vi "Read Roles.vi"(8 "error in (no error)":errorcluster, 11 "KickPenaltyAllyPlayVSS in":refnum<class "KickPenaltyAllyPlayVSS.lvclass">) -> (0 "error out":errorcluster, 2 "Roles":T1, 3 "KickPenaltyAllyPlayVSS out":refnum<class "KickPenaltyAllyPlayVSS.lvclass">)   [LabVIEW 2020, in "KickPenaltyAllyPlayVSS.lvclass"]
uses:
  KickPenaltyAllyPlayVSS.lvclass
  NormalAttackerRoleVSS_class/NormalAttackerRoleVSS.lvclass
  HaltRole_class/HaltRole.lvclass
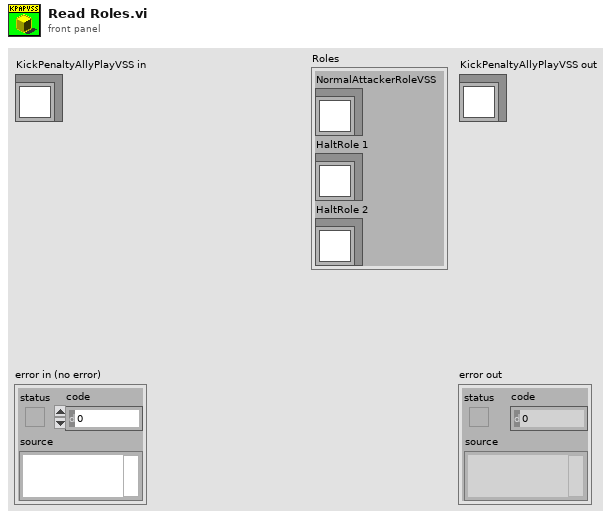
[diagram p1: front panel]
types:
  T1 = cluster{"NormalAttackerRoleVSS":refnum<class "NormalAttackerRoleVSS.lvclass">, "HaltRole 1":refnum<class "HaltRole.lvclass">, "HaltRole 2":refnum<class "HaltRole.lvclass">}
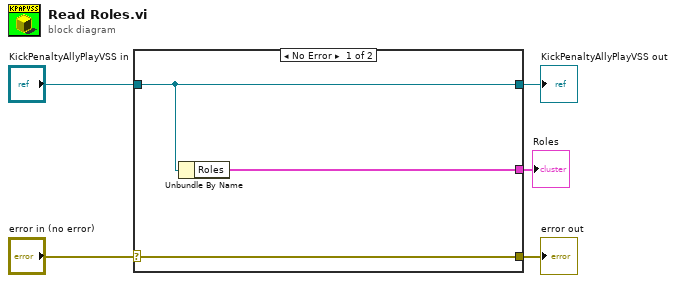
[diagram p0: block diagram]
diagram:
  n1 = case shown="No Error" "error in (no error)" {
    selector: "error in (no error)" -> [w8 w9]
    tunnel: [w8 w9] -> w4
    tunnel: [w7 w10] -> w2
    tunnel: "KickPenaltyAllyPlayVSS in" -> [w7 w10]
    tunnel: [w6 _] -> w1
    frame No Error {
      n2 = Unbundle By Name(w7) -> ("Roles"=w6:T1)
    }
    frame Error {
    }
  }
  "error out" <- w4
  "KickPenaltyAllyPlayVSS out" <- w2
  "Roles" <- w1
